vi "Agilent VNA Format Model String.vi"(1 "Model":string) -> (0 "Model":T1=enum."8753X")   [LabVIEW 2011]
uses:
  TypeDefs/Agilent VNA Model.ctl
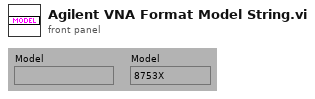
[diagram p1: front panel]
types:
  T1 = typedef "Agilent VNA Model.ctl" = enum16{"Not Supported", "8510X", "8719X", "8720X", "8722X", "8753X", "ENA", "PNA", "Field Fox"}
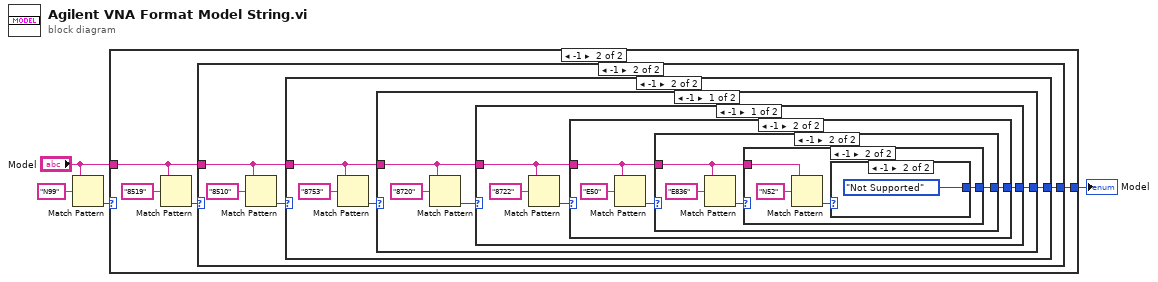
[diagram p0: block diagram]
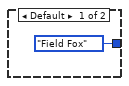
[diagram p2: hidden frame]
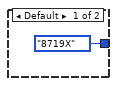
[diagram p3: hidden frame]
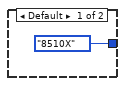
[diagram p4: hidden frame]
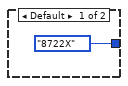
[diagram p5: hidden frame]
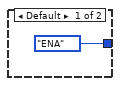
[diagram p6: hidden frame]
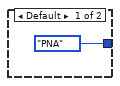
[diagram p7: hidden frame]
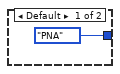
[diagram p8: hidden frame]
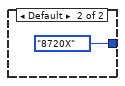
[diagram p9: hidden frame]
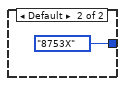
[diagram p10: hidden frame]
diagram:
  n1 = Match Pattern(string="Model", regular expression="N99") -> (offset past match=w1:i32)  [unwired: 4 out]
  n2 = case shown="-1" w1 {
    tunnel: [Agilent_VNA_Model."Field Fox" ("Model") w9] -> w4
    tunnel: "Model" -> [_ w6]
    frame Default {
    }
    frame -1 {
      n3 = Match Pattern(string=w6, regular expression="8519") -> (offset past match=w7:i32)  [unwired: 4 out]
      n4 = case shown="-1" w7 {
        tunnel: w6 -> [_ w12]
        tunnel: [Agilent_VNA_Model."8719X" ("Model") w11] -> w9
        frame Default {
        }
        frame -1 {
          n5 = Match Pattern(string=w12, regular expression="8510") -> (offset past match=w13:i32)  [unwired: 4 out]
          n6 = case shown="-1" w13 {
            tunnel: [Agilent_VNA_Model."8510X" ("Model") w17] -> w11
            tunnel: w12 -> [_ w16]
            frame Default {
            }
            frame -1 {
              n7 = Match Pattern(string=w16, regular expression="8753") -> (offset past match=w18:i32)  [unwired: 4 out]
              n8 = case shown="-1" w18 {
                tunnel: [w21 Agilent_VNA_Model."8753X" ("Model")] -> w17
                tunnel: w16 -> [w20 _]
                frame -1 {
                  n9 = Match Pattern(string=w20, regular expression="8720") -> (offset past match=w22:i32)  [unwired: 4 out]
                  n10 = case shown="-1" w22 {
                    tunnel: [w24 Agilent_VNA_Model."8720X" ("Model")] -> w21
                    tunnel: w20 -> [w25 _]
                    frame -1 {
                      n11 = Match Pattern(string=w25, regular expression="8722") -> (offset past match=w26:i32)  [unwired: 4 out]
                      n12 = case shown="-1" w26 {
                        tunnel: w25 -> [_ w30]
                        tunnel: [Agilent_VNA_Model."8722X" ("Model") w29] -> w24
                        frame Default {
                        }
                        frame -1 {
                          n13 = Match Pattern(string=w30, regular expression="E50") -> (offset past match=w31:i32)  [unwired: 4 out]
                          n14 = case shown="-1" w31 {
                            tunnel: w30 -> [_ w35]
                            tunnel: [Agilent_VNA_Model."ENA" ("Model") w34] -> w29
                            frame Default {
                            }
                            frame -1 {
                              n15 = Match Pattern(string=w35, regular expression="E836") -> (offset past match=w36:i32)  [unwired: 4 out]
                              n16 = case shown="-1" w36 {
                                tunnel: w35 -> [_ w41]
                                tunnel: [Agilent_VNA_Model."PNA" ("Model") w39] -> w34
                                frame Default {
                                }
                                frame -1 {
                                n17 = Match Pattern(string=w41, regular expression="N52") -> (offset past match=w40:i32)  [unwired: 4 out]
                                n18 = case shown="-1" w40 {
                                tunnel: [Agilent_VNA_Model."PNA" ("Model") Agilent_VNA_Model."Not Supported" ("Model")] -> w39
                                frame Default {
                                }
                                frame -1 {
                                }
                                }
                                }
                              }
                            }
                          }
                        }
                      }
                    }
                    frame Default {
                    }
                  }
                }
                frame Default {
                }
              }
            }
          }
        }
      }
    }
  }
  "Model" <- w4
